vi "TEMP RAMP (SubVI).vi"(0 "Device port":dbl=12.0, 1 "Numeric":i16, 2 "Tbyp":dbl, 3 "Numeric 2":i16, 4 "Seq":dbl[][](array[numeric])=[[20.0, 60.0, 40.0], [60.0, 40.0, 20.0], [100.0, 100.0, 100.0]], 5 "data":dynamicdata(waveform), 6 "bypass":i32, 9 "err":i32, 16 "Tfail":dbl) -> (7 "Sp - Tset":i32, 8 "T":dbl, 10 "Sp":dbl, 11 "Change":i32, 12 "tr":dbl, 13 "Debug msg":dbl, 14 "Elapsed":i32, 15 "Tset":dbl, 17 "Step":i32, 18 "Tinit":dbl, 19 "return type":dbl)   [LabVIEW 2015]
uses:
  BERTTA.dll
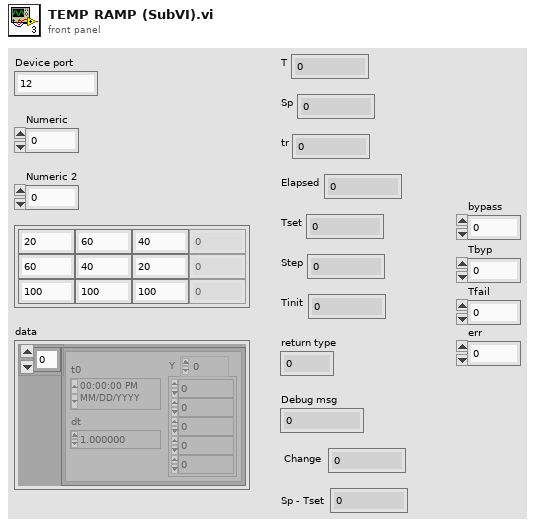
[diagram p1: front panel]
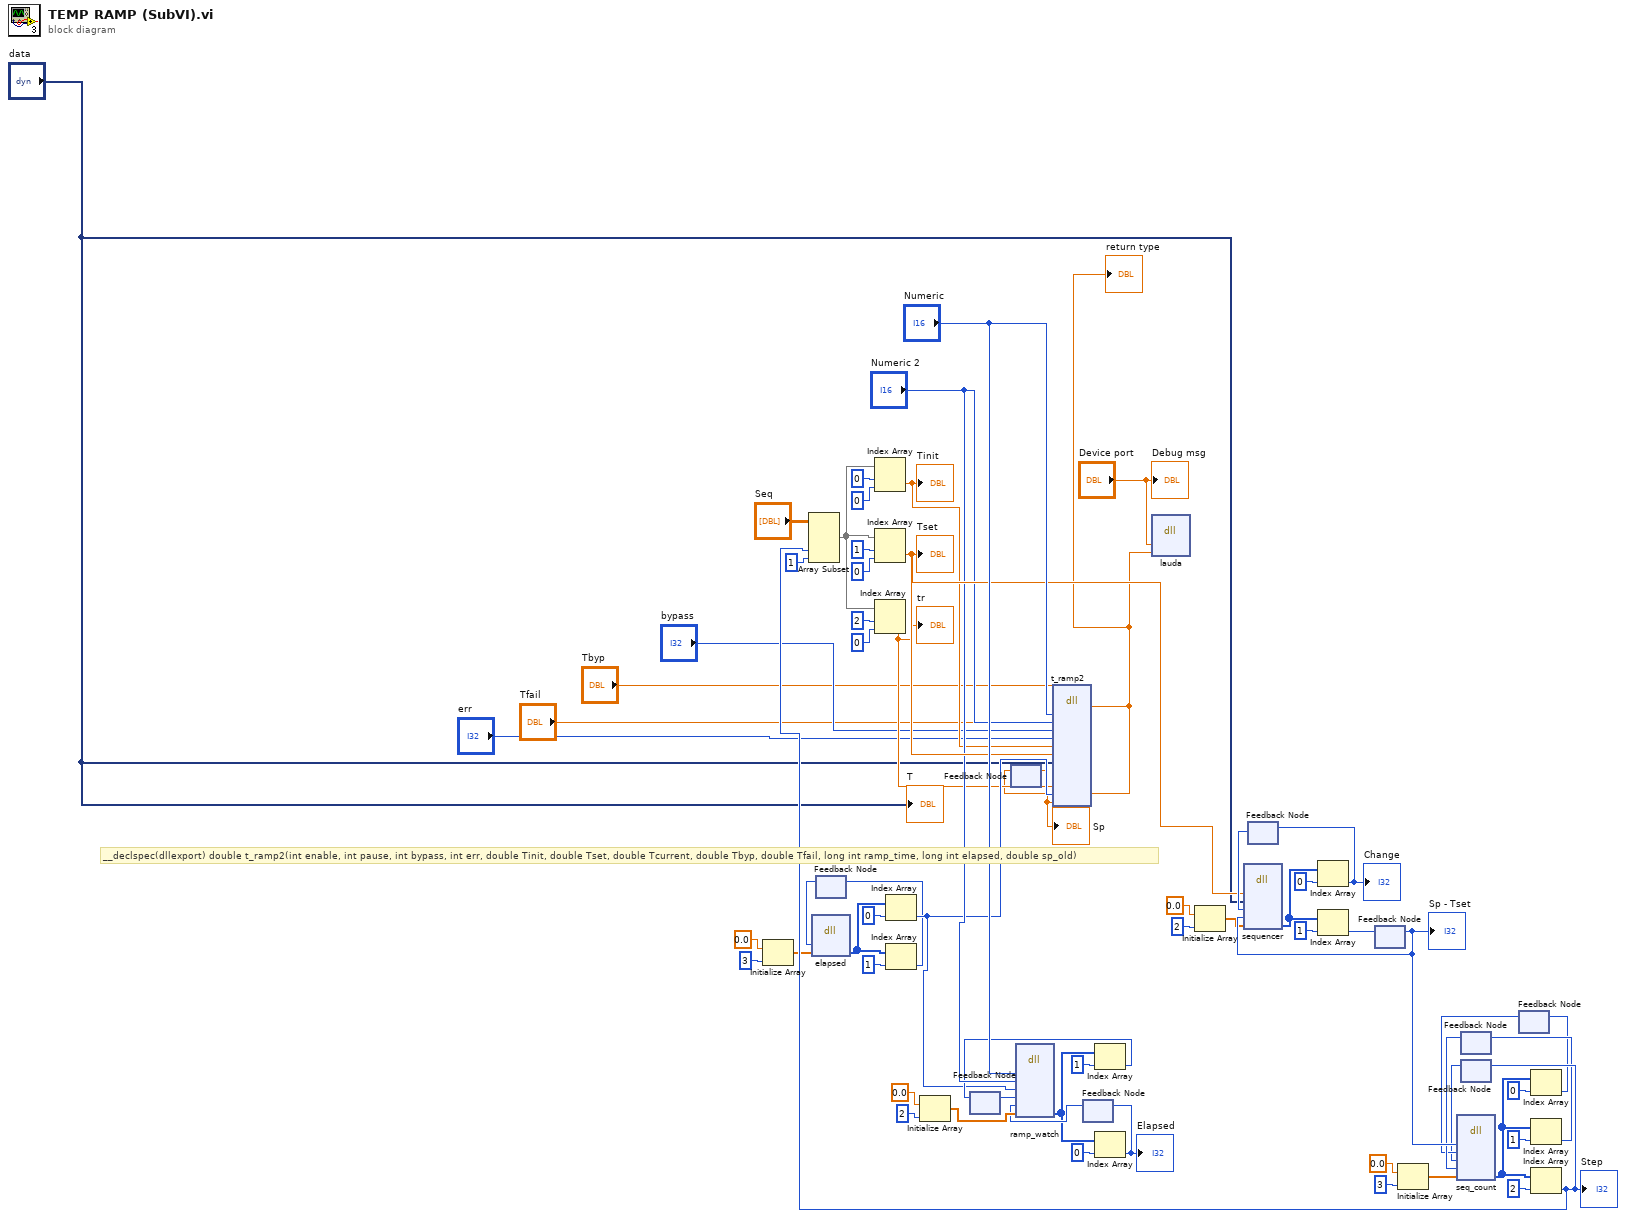
[diagram p0: block diagram]
diagram:
  # "__declspec(dllexport) double t_ramp2(int enable, int pause, int bypass, int err, double Tinit, double Tset, double Tcurrent, double Tbyp, double Tfail, long int ramp_time, long int elapsed, double sp_old)"
  n1 = Initialize Array(0.0 ("element"), 3 ("dimension size")) -> (w7:dbl[])
  n2 = feedback #1() -> (w13:i32)  [unwired: 1 in]
  n3 = dll-call lib="C:/Users/xlaraser/Documents/Visual Studio 2017/Projects/Bertta/BERTTA/Debug/BERTTA.dll" fn="elapsed"("last_time"=w13, "params"=w7) -> ("params"=w27:i32[])  [unwired: 5 in, 2 out]
  n4 = Index Array(array=w27, index=0) -> (element=w28:i32)
  n5 = Index Array(array=w27, index=1) -> (element=w12:i32)
  n6 = feedback-in #1(w12) -> ()
  n7 = Initialize Array(0.0 ("element"), 2 ("dimension size")) -> (w38:dbl[])
  n8 = feedback #2() -> (w35:i32)  [unwired: 1 in]
  n9 = feedback #3() -> (w6:dbl)  [unwired: 1 in]
  "Sp" <- w6
  n10 = feedback #4() -> (w33:i32)  [unwired: 1 in]
  n11 = dll-call lib="C:/Users/xlaraser/Documents/Visual Studio 2017/Projects/Bertta/BERTTA/Debug/BERTTA.dll" fn="ramp_watch"("enable"="Numeric", "pause"="Numeric 2", "elapsed"=w28, "elapsed_previous"=w35, "elapsed_total"=w33, "params"=w38) -> ("params"=w31:i32[])  [unwired: 9 in, 2 out]
  n12 = Index Array(array=w31, index=1) -> (element=w34:i32)
  n13 = feedback-in #2(w34) -> ()
  n14 = Index Array(array=w31, index=0) -> (element=w32:i32)
  "Elapsed" <- w32
  n15 = feedback-in #4(w32) -> ()
  n16 = Initialize Array(0.0 ("element"), 2 ("dimension size")) -> (w48:dbl[])
  n17 = feedback #5() -> (w45:i32)  [unwired: 1 in]
  n18 = feedback #6() -> (w62:i32)  [unwired: 1 in]
  "Sp - Tset" <- w62
  n19 = Initialize Array(0.0 ("element"), 3 ("dimension size")) -> (w50:dbl[])
  n20 = feedback #7() -> (w59:i32)  [unwired: 1 in]
  n21 = feedback #8() -> (w57:i32)  [unwired: 1 in]
  n22 = feedback #9() -> (w58:i32)  [unwired: 1 in]
  n23 = dll-call lib="C:/Users/xlaraser/Documents/Visual Studio 2017/Projects/Bertta/BERTTA/Debug/BERTTA.dll" fn="seq_count"("in1"=w62, "in2"=w58, "in3"=w57, "in4"=w59, "params"=w50) -> ("params"=w56:i32[])  [unwired: 8 in, 2 out]
  n24 = Index Array(array=w56, index=0) -> (element=w60:i32)
  n25 = feedback-in #9(w60) -> ()
  n26 = Index Array(array=w56, index=1) -> (element=w61:i32)
  n27 = feedback-in #7(w61) -> ()
  n28 = Index Array(array=w56, index=2) -> (element=w63:i32)
  "Step" <- w63
  n29 = Array Subset(array="Seq", index (col)=w63, length (col)=1 ("length")) -> (w21:dbl[][])  [unwired: 2 in]
  n30 = Index Array(array=w21, index (row)=0, index (col)=0 ("disabled index (col)")) -> (element=w22:dbl)
  "Tinit" <- w22
  n31 = Index Array(array=w21, index (row)=1, index (col)=0 ("disabled index (col)")) -> (element=w40:dbl)
  "Tset" <- w40
  n32 = Index Array(array=w21, index (row)=2, index (col)=0 ("disabled index (col)")) -> (element=w26:dbl)
  "tr" <- w26
  n33 = dll-call lib="C:/Users/xlaraser/Documents/Visual Studio 2017/Projects/Bertta/BERTTA/Debug/BERTTA.dll" fn="t_ramp2"("enable"="Numeric", "pause"="Numeric 2", "bypass"="bypass", "err"="err", "Tinit"=w22, "Tset"=w40, "Tcurrent"="data", "Tbyp"="Tbyp", "Tfail"="Tfail", "ramp_time"=w26, "elapsed"=w28, "sp_old"=w6) -> ("return type"=w15:dbl)  [unwired: 15 in, 2 out]
  "return type" <- w15
  n34 = feedback-in #3(w15) -> ()
  n35 = dll-call lib="C:/Users/xlaraser/Documents/Visual Studio 2017/Projects/Bertta/BERTTA/Debug/BERTTA.dll" fn="lauda"("port"="Device port", "set_temp"=w15) -> ()  [unwired: 6 in, 2 out]
  n36 = dll-call lib="C:/Users/xlaraser/Documents/Visual Studio 2017/Projects/Bertta/BERTTA/Debug/BERTTA.dll" fn="sequencer"("Tset"=w40, "Tcurrent"="data", "treshold"=w45, "seq_previous"=w62, "params"=w48) -> ("params"=w43:i32[])  [unwired: 8 in, 2 out]
  n37 = Index Array(array=w43, index=0) -> (element=w44:i32)
  "Change" <- w44
  n38 = feedback-in #5(w44) -> ()
  n39 = Index Array(array=w43, index=1) -> (element=w49:i32)
  n40 = feedback-in #6(w49) -> ()
  n41 = feedback-in #8(w63) -> ()
  "T" <- "data"
  "Debug msg" <- "Device port"
